vi "AB_ChangeSharedLibExtension.vi"(8 "error in (no error)":errorcluster, 10 "Target OS":T1(ring), 11 "Target file name":string) -> (0 "error out":errorcluster, 3 "New target file name":string)   [LabVIEW 2020]
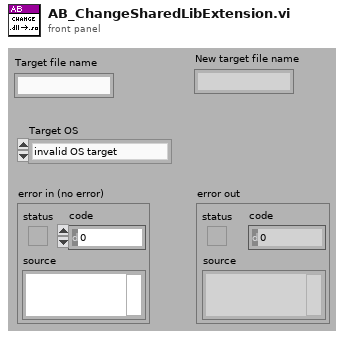
[diagram p1: front panel]
types:
  T1 = enum32{"invalid OS target", "Mac OS", "Windows 3.1", "Windows 95/NT", "Solaris 1", "Solaris 2", "HP-UX", "PowerMAX", "Linux", "Irix", "Rhapsody", "BeOS", "AIX", "OSF1", "VxWorks", "PharLap", "Carbon", "RTX", "Windows x64", "Linux x64", "Mac OS X x64"}
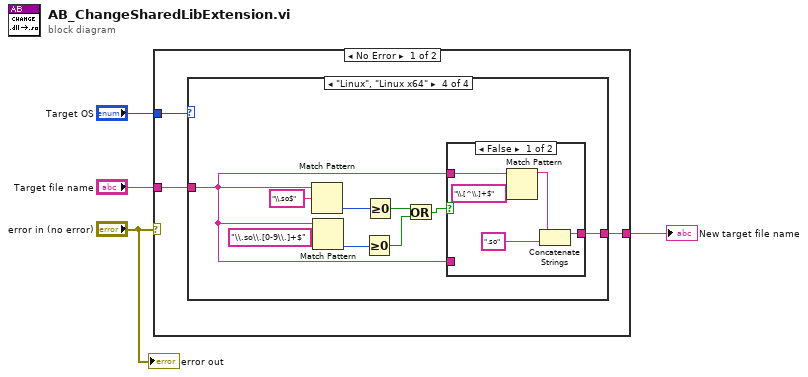
[diagram p0: block diagram]
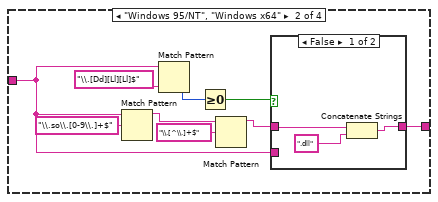
[diagram p3: hidden frame]
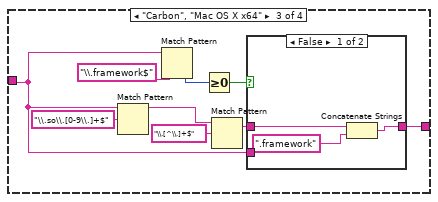
[diagram p5: hidden frame]
diagram:
  n1 = case shown="No Error" "error in (no error)" {
    tunnel: [w7 w50] -> w4
    tunnel: "Target file name" -> [w6 w50]
    tunnel: "Target OS" -> [w5 _]
    frame No Error {
      n2 = case shown="\"Linux\", \"Linux x64\"" w5 {
        tunnel: w6 -> [w8 w11 w23 w35]
        tunnel: [w8 w17 w30 w43] -> w7
        frame Default {
        }
        frame "Windows 95/NT", "Windows x64" {
          n3 = Match Pattern(string=w11, regular expression="\\.so\\.[0-9\\.]+$") -> (before substring=w10:string)  [unwired: 1 in, 3 out]
          n4 = Match Pattern(string=w11, regular expression="\\.[Dd][Ll][Ll]$") -> (offset past match=w13:i32)  [unwired: 1 in, 3 out]
          n5 = Greater Or Equal To 0?(x=w13) -> (x >= 0?=w12:bool)
          n6 = Match Pattern(string=w10, regular expression="\\.[^\\.]+$") -> (before substring=w16:string)  [unwired: 1 in, 3 out]
          n7 = case shown="False" w12 {
            tunnel: w16 -> [w18 _]
            tunnel: [w19 w21] -> w17
            tunnel: w11 -> [_ w21]
            frame False {
              n8 = Concatenate Strings(w18, ".dll" ("y")) -> (w19:string)
            }
            frame True {
            }
          }
        }
        frame "Carbon", "Mac OS X x64" {
          n9 = Match Pattern(string=w23, regular expression="\\.so\\.[0-9\\.]+$") -> (before substring=w22:string)  [unwired: 1 in, 3 out]
          n10 = Match Pattern(string=w23, regular expression="\\.framework$") -> (offset past match=w26:i32)  [unwired: 1 in, 3 out]
          n11 = Greater Or Equal To 0?(x=w26) -> (x >= 0?=w29:bool)
          n12 = Match Pattern(string=w22, regular expression="\\.[^\\.]+$") -> (before substring=w25:string)  [unwired: 1 in, 3 out]
          n13 = case shown="False" w29 {
            tunnel: w25 -> [w31 _]
            tunnel: [w32 w34] -> w30
            tunnel: w23 -> [_ w34]
            frame False {
              n14 = Concatenate Strings(w31, ".framework" ("y")) -> (w32:string)
            }
            frame True {
            }
          }
        }
        frame "Linux", "Linux x64" {
          n15 = Match Pattern(string=w35, regular expression="\\.so$") -> (offset past match=w41:i32)  [unwired: 1 in, 3 out]
          n16 = Match Pattern(string=w35, regular expression="\\.so\\.[0-9\\.]+$") -> (offset past match=w38:i32)  [unwired: 1 in, 3 out]
          n17 = Greater Or Equal To 0?(x=w38) -> (x >= 0?=w36:bool)
          n18 = Greater Or Equal To 0?(x=w41) -> (x >= 0?=w40:bool)
          n19 = Or(x=w40, y=w36) -> (x .or. y?=w37:bool)
          n20 = case shown="False" w37 {
            tunnel: [w47 w49] -> w43
            tunnel: w35 -> [_ w49]
            tunnel: w35 -> [w45 _]
            frame False {
              n21 = Match Pattern(string=w45, regular expression="\\.[^\\.]+$") -> (before substring=w44:string)  [unwired: 1 in, 3 out]
              n22 = Concatenate Strings(w44, ".so" ("y")) -> (w47:string)
            }
            frame True {
            }
          }
        }
      }
    }
    frame Error {
    }
  }
  "New target file name" <- w4
  "error out" <- "error in (no error)"
